vi "Packet Time Alignment.vi"(8 "packet start index valid":bool=TRUE, 9 "packet start index":u16, 10 "sample in valid":bool=TRUE, 11 "channels in":T1) -> (1 "packet start":bool=TRUE, 2 "output valid":bool=TRUE, 3 "channels out":T1)   [LabVIEW 2020]
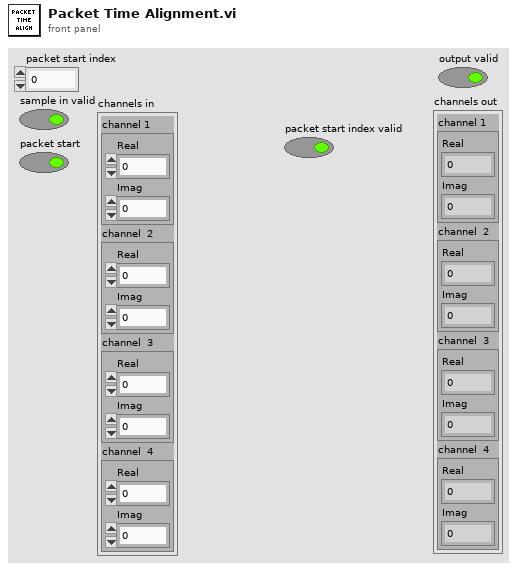
[diagram p1: front panel]
types:
  T1 = cluster{"channel 1 ":cluster{"Real":fxp<+/-,16,3>, "Imag":fxp<+/-,16,3>}, "channel  2":cluster{"Real":fxp<+/-,16,3>, "Imag":fxp<+/-,16,3>}, "channel  3":cluster{"Real":fxp<+/-,16,3>, "Imag":fxp<+/-,16,3>}, "channel  4":cluster{"Real":fxp<+/-,16,3>, "Imag":fxp<+/-,16,3>}}
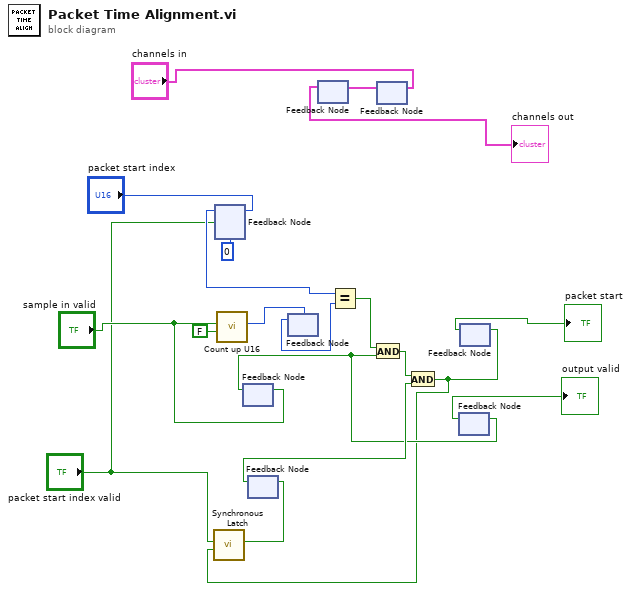
[diagram p0: block diagram]
diagram:
  n1 = feedback-in #1("packet start index", "packet start index valid") -> ()
  n2 = feedback #1(u16 0 ("packet start index")) -> (w13:u16)
  n3 = call "Count up U16.vi"("reset"=FALSE, "increment"="sample in valid") -> ("count out"=w14:u16)  [unwired: 9 in]
  n4 = feedback #2() -> (w7:bool)  [unwired: 1 in]
  n5 = feedback-in #2("sample in valid") -> ()
  n6 = feedback #3() -> (w9:bool)  [unwired: 1 in]
  n7 = feedback #4() -> (w12:u16)  [unwired: 1 in]
  n8 = feedback-in #4(w14) -> ()
  n9 = feedback #5() -> (→"channels out":T1)  [unwired: 1 in]
  n10 = Equal?(x=w13, y=w12) -> (x = y?=w6:bool)
  n11 = And(x=w6, y=w7) -> (x .and. y?=w10:bool)
  n12 = feedback #6() -> (w19:T1)  [unwired: 1 in]
  n13 = feedback-in #5(w19) -> ()
  n14 = feedback-in #6("channels in") -> ()
  n15 = And(x=w10, y=w9) -> (x .and. y?=w2:bool)
  n16 = call "Synchronous Latch.vi"("clear"=w2, "set"="packet start index valid") -> ("out"=w3:bool)  [unwired: 9 in]
  n17 = feedback-in #3(w3) -> ()
  n18 = feedback #7() -> (→"output valid":bool)  [unwired: 1 in]
  n19 = feedback-in #7(w7) -> ()
  n20 = feedback #8() -> (→"packet start":bool)  [unwired: 1 in]
  n21 = feedback-in #8(w2) -> ()
